vi "Flywheel_Set.vi"   [LabVIEW 2020]
uses:
  Globals/Flywheel_Globals.vi
  Flywheel_States.ctl
  Robot Global Data.vi
  <vilib>/Rock Robotics/WPI/DriverStation/WPI_DriverStationRobotMode2.ctl
  Flywheel_Cluster.ctl
types:
  T1 = typedef "Flywheel_Cluster.ctl" = cluster{"Flywheel_Throttle":dbl, "Control_States":T2, "Auto_Speed":bool, "Flywheel_On":bool, "Parameter_1":dbl, "Parameter_2":dbl, "Auto_Notifier":refnum<notifier>, "Step":dbl}
  T2 = typedef "Flywheel_States.ctl" = enum16{"No-Op", "Percent_Voltage", "Speed_Control_Manual", "Speed_Control_Auto", "Command_SpinUp", "Command_SpinUpAuto"}
  T3 = typedef "WPI_DriverStationRobotMode2.ctl" = enum16{"Autonomous Disabled", "Autonomous Enabled", "Teleop Disabled", "Teleop Enabled", "Disconnected", "Finish", "Test Disabled", "Test Enabled", "Emergency Stopped"}
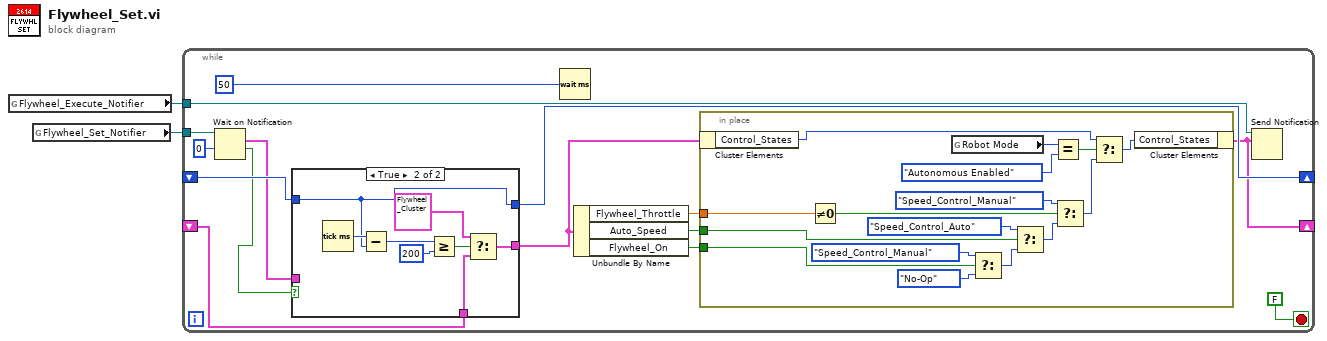
[diagram p0: block diagram]
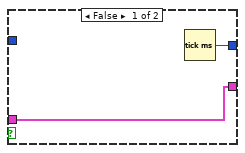
[diagram p2: hidden frame]
diagram:
  n1 = global read "Flywheel_Globals.vi" "Flywheel_Execute_Notifier"() -> (w1:refnum<notifier>)
  n2 = global read "Flywheel_Globals.vi" "Flywheel_Set_Notifier"() -> (w2:refnum<notifier>)
  n3 = while {
    tunnel: w2 -> [w17]
    tunnel: w1 -> [w13]
    shift-right: [w4] -> _
    shift-left: _ -> [w3]
    shift-right: [w9] -> _
    shift-left: _ -> [w8]
    stop <- FALSE stop-if-true
    n4 = Wait on Notification(notifier=w17, timeout in ms (-1)=0) -> (notification=w5:T1, timed out?=w7:bool)  [unwired: 2 in, 2 out]
    n5 = case shown="True" w7 {
      tunnel: w5 -> [w19 _]
      tunnel: [w19 w22] -> w10
      tunnel: [w18 w26] -> w9
      tunnel: w8 -> [_ w26]
      tunnel: w3 -> [_ w20]
      frame False {
        n6 = Tick Count (ms)() -> (millisecond timer value=w18:u32)
      }
      frame True {
        n7 = Tick Count (ms)() -> (millisecond timer value=w27:u32)
        n8 = Subtract(x=w27, y=w26) -> (x-y=w25:u32)
        n9 = Greater Or Equal?(x=w25, y=u32 200) -> (x >= y?=w23:bool)
        n10 = Select(t=T1 {"Flywheel_Throttle"=0.0, "Control_States"=enum."No-Op", "Auto_Speed"=FALSE, "Flywheel_On"=FALSE, "Parameter_1"=0.0, "Parameter_2"=0.0, "Auto_Notifier"=refnum, "Step"=0.0} ("Flywheel_Cluster"), s=w23, f=w20) -> (s? t:f=w22:T1)
      }
    }
    n11 = Wait (ms)(milliseconds to wait=u32 50) -> ()  [unwired: 1 out]
    n12 = Unbundle By Name(w10) -> ("Flywheel_Throttle"=w16:dbl, "Auto_Speed"=w14:bool, "Flywheel_On"=w15:bool)
    n13 = in-place {
      in-place-border: w16 -> [w43]
      in-place-border: w15 -> [w42]
      in-place-border: w14 -> [w34]
      n14 = in-place-cluster #1(w10) -> ("Control_States"=w28:T2)
      n15 = Not Equal To 0?(x=w43) -> (x != 0?=w36:bool)
      n16 = global read "Robot Global Data.vi" "Robot Mode"() -> (w31:T3)
      n17 = Select(t=Flywheel_States."Speed_Control_Manual" ("Control_States"), s=w42, f=Flywheel_States."No-Op" ("Control_States")) -> (s? t:f=w41:T2)
      n18 = Select(t=Flywheel_States."Speed_Control_Auto" ("Control_States"), s=w34, f=w41) -> (s? t:f=w37:T2)
      n19 = Equal?(x=w31, y=WPI_DriverStationRobotMode2."Autonomous Enabled") -> (x = y?=w29:bool)
      n20 = Select(t=Flywheel_States."Speed_Control_Manual" ("Control_States"), s=w36, f=w37) -> (s? t:f=w33:T2)
      n21 = Select(t=w28, s=w29, f=w33) -> (s? t:f=w32:T2)
      n22 = in-place-cluster #1("Control_States"=w32) -> (w4:T1)
    }
    n23 = Send Notification(notification=w4, notifier=w13) -> ()  [unwired: 1 in, 2 out]
  }
